vi "Show bars.vi"() -> ()   [LabVIEW 2012]
uses:
  Bar info.ctl
  <vilib>/Platform/TimedLoop/XDataNode/timing_clust.ctl
  <vilib>/Platform/TimedLoop/XDataNode/nitl_modes.ctl
  <vilib>/Platform/TimedLoop/XDataNode/wakeup.ctl
  <vilib>/platform/TimedLoop/XDataNode/XDataNode.xnode
  <vilib>/Platform/TimedLoop/XDataNode/XDNodeRunTimeDep.lvlib
panel:
  out "Bars":picture
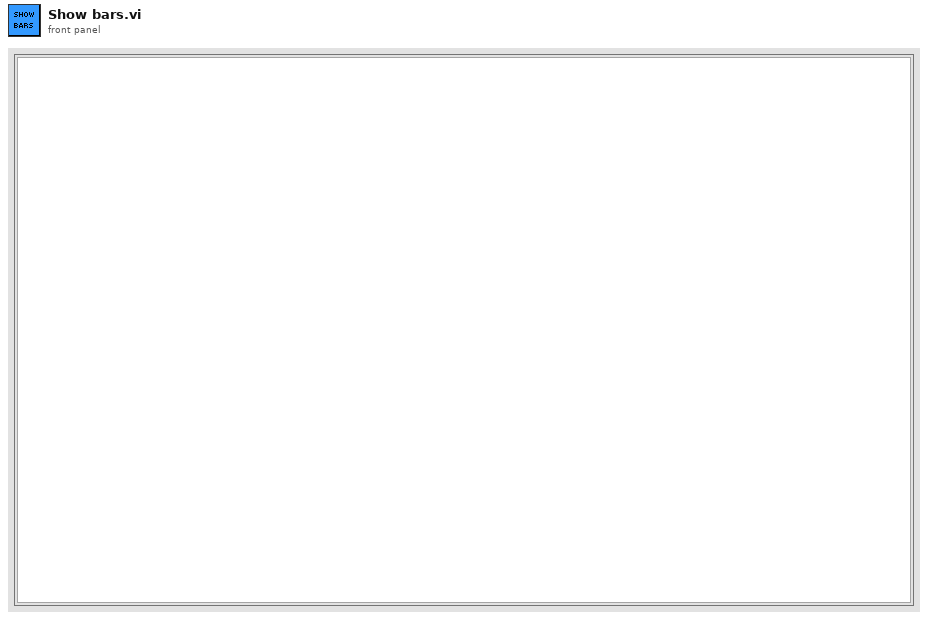
[diagram p1: front panel]
types:
  T1 = typedef "Bar info.ctl" = cluster{"Bar width":dbl, "Bar speed":dbl, "Amplitude":dbl, "Frequency":dbl, "Contrast":dbl, "Refresh rate":dbl, "Monitor scale":dbl, "Command":enum16{"Go", "Stop", "Quit"}}
  T2 = typedef "XDNodeRunTimeDep.lvlib/timing_clust.ctl" = cluster{"Expected End [f-1]":u64, "Actual End [f-1]":u64, "Finished Late? [f-1]":bool, "Expected End [i-1]":u64, "Actual End [i-1]":u64, "Finished Late? [i-1]":bool, "Expected Start [i]":u64, "Actual Start [i]":u64, "Expected Start [f]":u64, "Actual Start [f]":u64, "Source Name":string, "Structure Name":string, "Period":i64, "Deadline":i64, "Offset":i64, "Start":i64, "Priority":i32, "Timeout":i32, "Mode":T3, "Wakeup Reason":T4, "Error":errorcluster, "Source Type":string, "Secondary Source Type":string, "Global End Time":u64, "Global Start Time":u64, "Frame Duration":u64, "Iteration Duration":u64, "Assigned CPU":i32, "I/O Scan Engine Mode":u32}
  T3 = typedef "XDNodeRunTimeDep.lvlib/nitl_modes.ctl" = enum32{"No Change", "Process missed periods, maintain original phase", "Discard missed periods, maintain original phase", "Process missed periods, ignore original phase", "Discard missed periods, ignore original phase"}
  T4 = typedef "XDNodeRunTimeDep.lvlib/wakeup.ctl" = enum32{"Normal", "Aborted", "Asynchronous wakeup", "Timing source error", "Timed loop error", "Timeout"}
  T5 = typedef "LVBoundsTypeDef.ctl" = cluster{"Width":u32, "Height":u32}
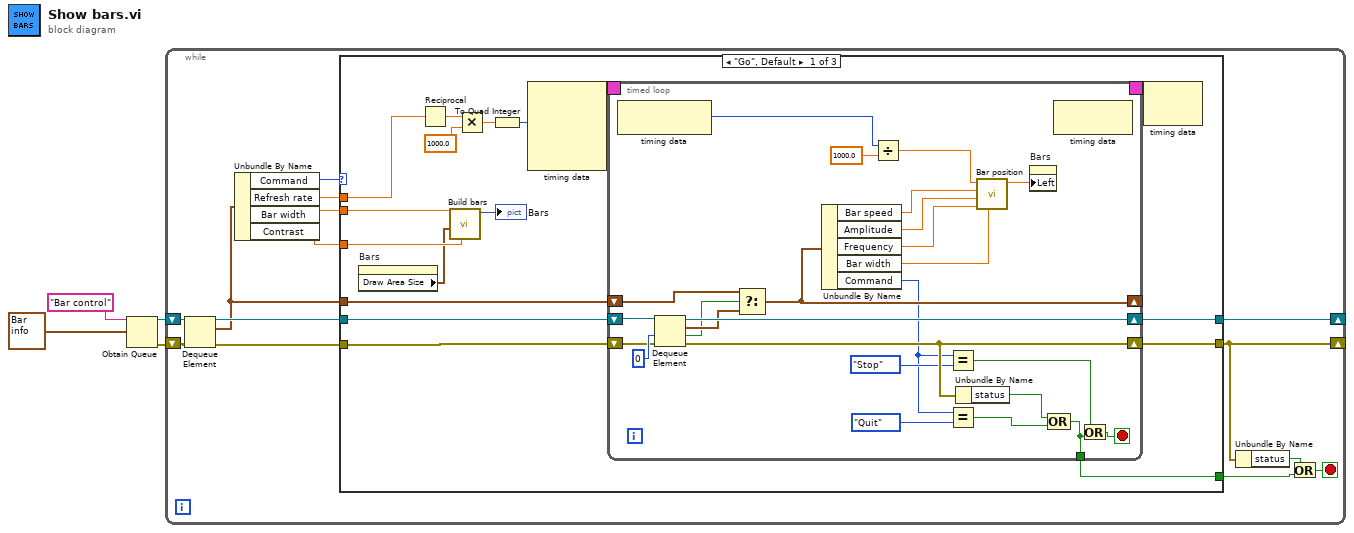
[diagram p0: block diagram]
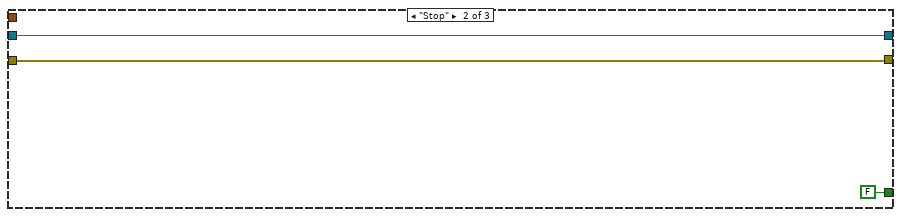
[diagram p2: hidden frame]
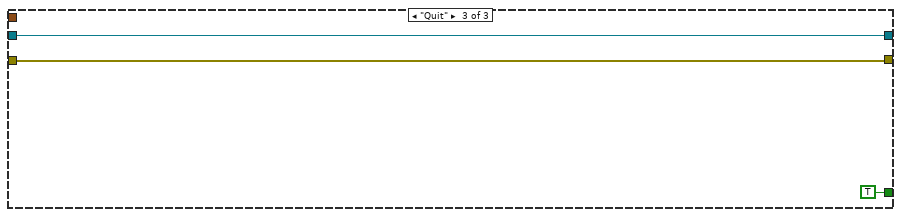
[diagram p3: hidden frame]
diagram:
  n1 = Obtain Queue(name (unnamed)="Bar control", element data type=T1 {"Bar width"=2.0, "Bar speed"=10.0, "Amplitude"=0.0, "Frequency"=0.0, "Contrast"=1.0, "Refresh rate"=0.0, "Monitor scale"=40.0, "Command"=enum."Stop"} ("Bar info")) -> (queue out=w1:refnum<queue>, error out=w2:errorcluster)  [unwired: 3 in, 1 out]
  n2 = while {
    shift-right: [w14] -> _
    shift-left: w1 -> [w17]
    shift-right: [w8] -> _
    shift-left: w2 -> [w18]
    stop <- w5 stop-if-true
    n3 = Dequeue Element(queue=w17, error in (no error)=w18) -> (queue out=w16:refnum<queue>, element=w9:T1, error out=w15:errorcluster)  [unwired: 1 in, 1 out]
    n4 = Unbundle By Name(w9) -> ("Command"=w11:enum16{"Go", "Stop", "Quit"}, "Refresh rate"=w10:dbl, "Bar width"=w13:dbl, "Contrast"=w12:dbl)
    n5 = case shown="\"Go\", Default" w11 {
      tunnel: w16 -> [w33 w70 w73]
      tunnel: w15 -> [w32 w69 w72]
      tunnel: [w31 w69 w72] -> w8
      tunnel: [w30 w70 w73] -> w14
      tunnel: w13 -> [w29 _ _]
      tunnel: w12 -> [w28 _ _]
      tunnel: w10 -> [w20 _ _]
      tunnel: [w25 FALSE TRUE] -> w7
      tunnel: w9 -> [w24 _ _]
      frame "Go", Default {
        n6 = property on="Bars" class="Pict"() -> ("Draw Area Size"=w26:T5)  [unwired: 2 in, 2 out]
        n7 = Reciprocal(x=w20) -> (1/x=w23:dbl)
        n8 = call "Build bars.vi"("Contrast"=w28, "Draw Area Size"=w26, "Bar width (pix)"=w29) -> ("bars"=→"Bars":picture)  [unwired: 8 in]
        n9 = Multiply(x=w23, y=1000.0) -> (x*y=w21:dbl)
        n10 = To Quad Integer(1:w21) -> (0:w19:i64)
        n11 = node-c288(w19) -> (w35:T2)  [unwired: 3 in]
        n12 = timed-loop {
          timing: w35 -> [_]
          timing-out: [_] -> w34
          shift-right: [w45] -> _
          shift-left: w24 -> [w48]
          shift-right: [w51] -> w30
          shift-left: w33 -> [w53]
          shift-right: [w44] -> w31
          shift-left: w32 -> [w50]
          tunnel: [w36] -> w25
          stop <- w38 stop-if-true
          n13 = node-c288() -> (w60:i64)  [unwired: 1 in]
          n14 = Dequeue Element(queue=w53, timeout in ms (-1)=0, error in (no error)=w50) -> (queue out=w51:refnum<queue>, element=w47:T1, timed out?=w46:bool, error out=w44:errorcluster)
          n15 = Select(t=w48, s=w46, f=w47) -> (s? t:f=w45:T1)
          n16 = Unbundle By Name(w45) -> ("Bar speed"=w57:dbl, "Amplitude"=w56:dbl, "Frequency"=w55:dbl, "Bar width"=w54:dbl, "Command"=w41:enum16{"Go", "Stop", "Quit"})
          n17 = Divide(x=w60, y=1000.0) -> (x/y=w58:dbl)
          n18 = Equal?(x=w41, y=enum16{"Go", "Stop", "Quit"}."Stop" ("Command")) -> (x = y?=w37:bool)
          n19 = Equal?(x=w41, y=enum16{"Go", "Stop", "Quit"}."Quit" ("Command")) -> (x = y?=w49:bool)
          n20 = Unbundle By Name(w44) -> ("status"=w43:bool)
          n21 = call "Bar position.vi"("bar width (pix)"=w54, "frequency (Hz)"=w55, "amplitude (pix/s)"=w56, "speed (pix/s)"=w57, "time (s)"=w58) -> ("position out"=w39:dbl)  [unwired: 6 in]
          n22 = property on="Bars" class="Pict"("Left"=w39) -> ()  [unwired: 2 in, 2 out]
          n23 = Compound Arithmetic op=OR(w43, w49) -> (w36:bool)
          n24 = node-c288() -> ()  [unwired: 1 in, 1 out]
          n25 = Or(x=w37, y=w36) -> (x .or. y?=w38:bool)
        }
        n26 = node-c288(w34) -> ()  [unwired: 1 out]
      }
      frame "Stop" {
      }
      frame "Quit" {
      }
    }
    n27 = Unbundle By Name(w8) -> ("status"=w6:bool)
    n28 = Or(x=w6, y=w7) -> (x .or. y?=w5:bool)
  }
